vi "Initialize.vi"(8 "error in (no error)":errorcluster, 10 "Transform Attribute String":string, 11 "TransformTokenizer in":refnum<class "TransformTokenizer.lvclass">) -> (0 "error out":errorcluster, 3 "TransformTokenizer out":refnum<class "TransformTokenizer.lvclass">)   [LabVIEW 2019, in "TransformTokenizer.lvclass"]
uses:
  TransformTokenizer.lvclass
  TransformTokenizer.lvclass/TransformTokenizer.ctl
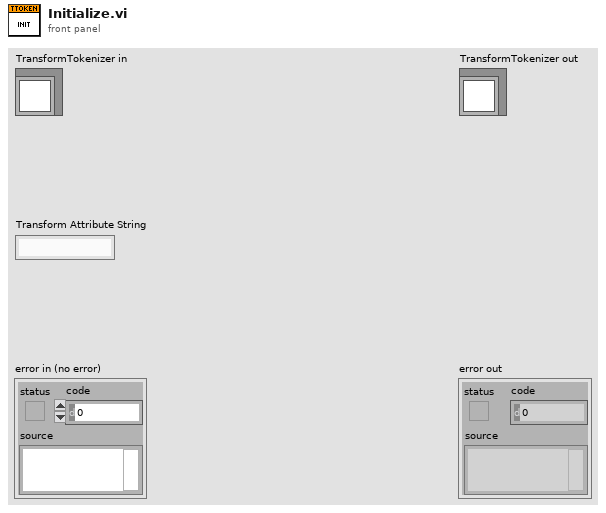
[diagram p1: front panel]
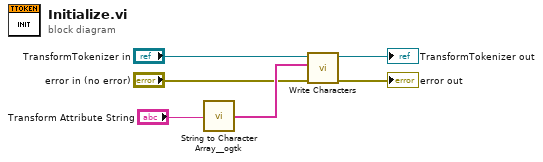
[diagram p0: block diagram]
diagram:
  n1 = call <userlib>:"String to Character Array__ogtk.vi"("Input String"="Transform Attribute String") -> ("Character Array"=w3:string[])
  n2 = call "Write Characters.vi"("error in (no error)"="error in (no error)", "Characters"=w3, "TransformTokenizer in"="TransformTokenizer in") -> ("error out"=→"error out":errorcluster, "TransformTokenizer out"=→"TransformTokenizer out":refnum<class "TransformTokenizer.lvclass">)  [unwired: 7 in]
